vi "OrdenarPosZagueiros.vi"(9 "geometry":T1, 11 "IA State Input 2":T2={"our_robots"=[], "enemy_robots"=[], "balls"=[], "geometry"={"line_width"=0, "field_length"=0, "field_width"=0, "boundary_width"=0, "referee_width"=0, "goal_width"=0, "goal_depth"=0, "goal_wall_width"=0, "center_circle_radius"=0, "defense_radius"=0, "defense_stretch"=0, "free_kick_from_defense_dist"=0, "penalty_spot_from_field_line_dist"=0, "penalty_line_from_spot_dist"=0}, "IA Judge"={"stage"="", "command"="", "our_goalie_id"=0.0, "enemy_goalie_id"=0.0, "command enum"=enum."Halt", "Time"=enum."Azul"}, "Received Timestamp"=timestamp(0 s since 1904-01-01), "Events"={"Touch"=FALSE, "Ball out"=FALSE, "id touch"=0.0, "Ball out of \nVision"=FALSE, "Ball inside \nGoalie area"=FALSE, "Robot not responding"=FALSE, "Robots responding status"=[1.0, 1.0, 1.0, 1.0, 1.0, 1.0], "Enemy Ball \nPossession"=FALSE, "Pass State"=FALSE, "id end of pass"=0.0, "Kick"=FALSE, "Id ini Possession"=0.0, "Ball Possesion"=FALSE, "Id Possesion"=0.0}}) -> (1 "Pos ordenana zagueiro 3":dbl[](array[numeric]) format="%#_13g", 2 "Pos ordenana zagueiro 2":dbl[](array[numeric]) format="%#_13g", 3 "Pos ordenana zagueiro 1":dbl[](array[numeric]) format="%#_13g")   [LabVIEW 2017]
uses:
  Core/AI Input.ctl
  Core/AI Robot.ctl
  Functions Enum.ctl
  AttackerStates.ctl
  Path Planning/RRT/PathDests.ctl
  Path Planning/RRT/PathDest.ctl
  Core/AI Ball.ctl
  Core/Field Size.ctl
  Core/AI Judge.ctl
  Command Enum.ctl
  Util/Events/Events.ctl
  b2e2cdbb-412d-44fb-bdeb-310cb0e881f7.vi
  75349cc0-a444-4d38-b1df-a3230ebe8c70.vi
  <vilib>/Array/Sort 2D Array - Pop Stack.vi
  <vilib>/Array/Sort 2D Array - Push Stack.vi
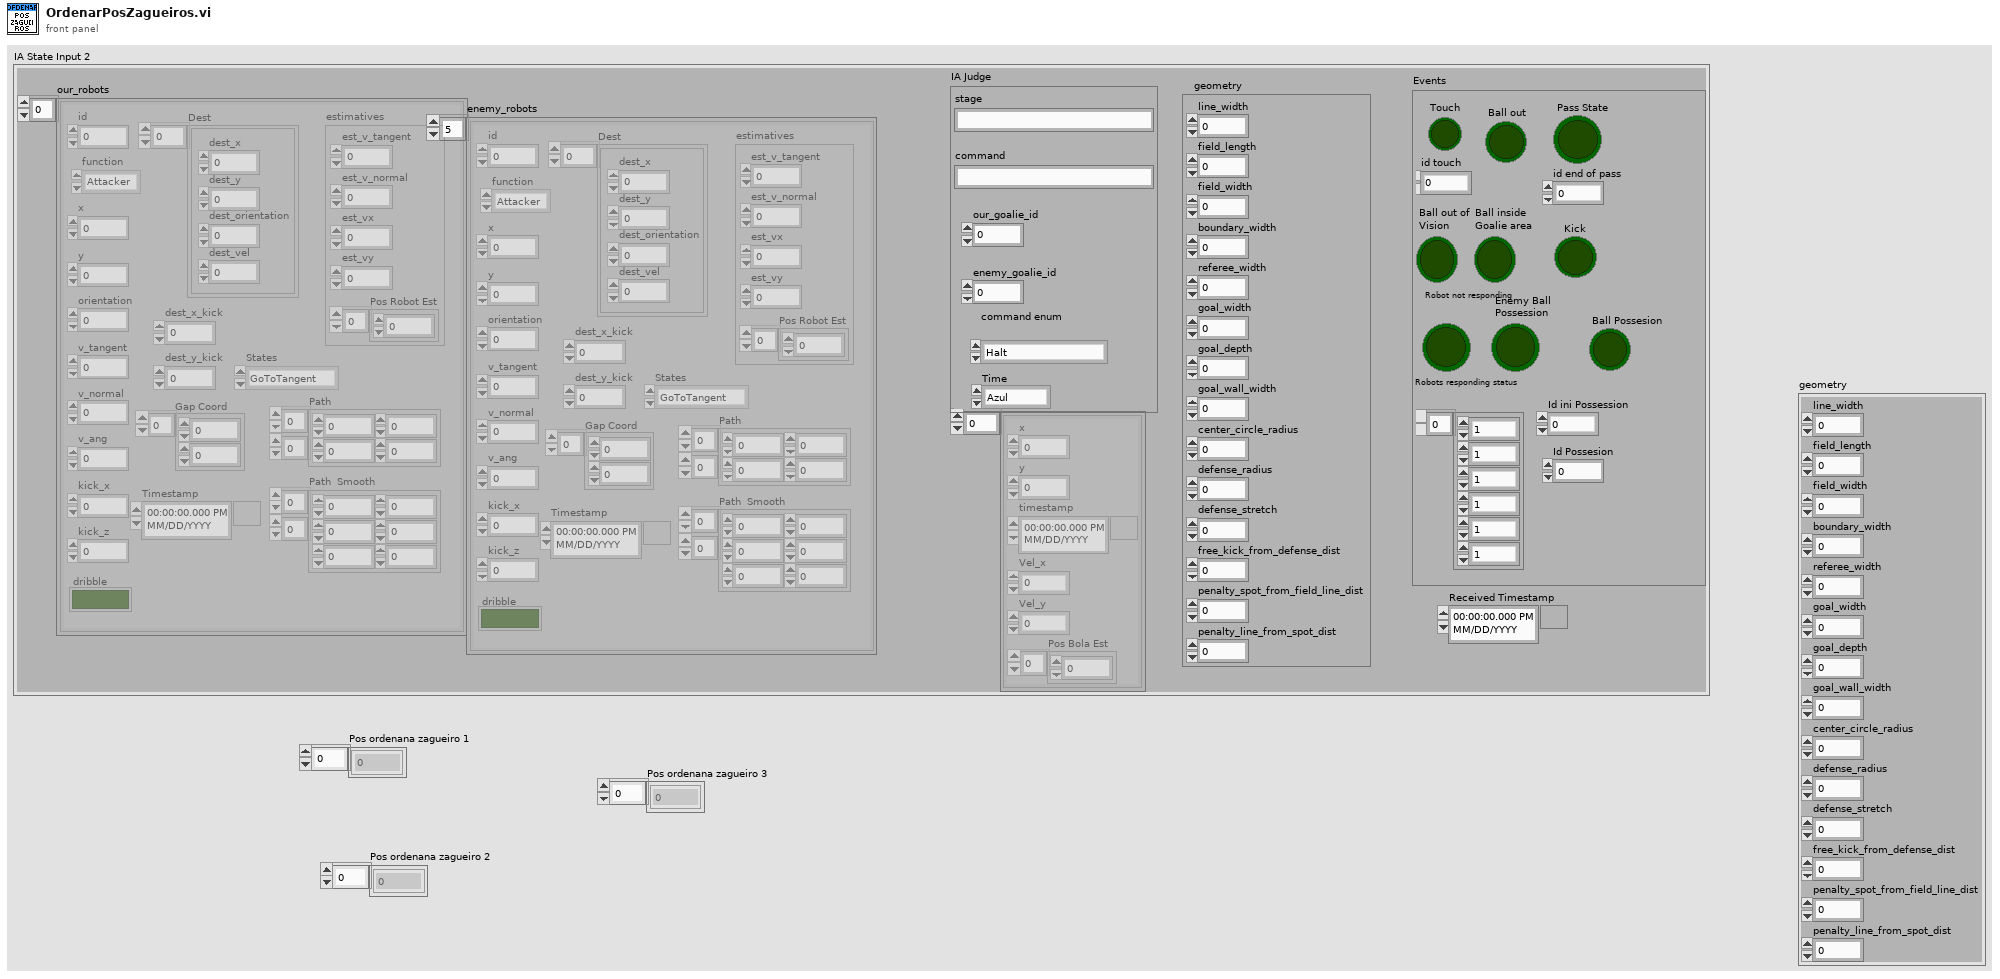
[diagram p1: front panel]
types:
  T1 = typedef "Field Size.ctl" = cluster{"line_width":u32, "field_length":u32, "field_width":u32, "boundary_width":u32, "referee_width":u32, "goal_width":u32, "goal_depth":u32, "goal_wall_width":u32, "center_circle_radius":u32, "defense_radius":u32, "defense_stretch":u32, "free_kick_from_defense_dist":u32, "penalty_spot_from_field_line_dist":u32, "penalty_line_from_spot_dist":u32}
  T2 = typedef "AI Input.ctl" = cluster{"our_robots":T3[], "enemy_robots":T3[], "balls":T8[], "geometry":T1, "IA Judge":T9, "Received Timestamp":timestamp, "Events":T11}
  T3 = typedef "AI Robot.ctl" = cluster{"id":u32, "function":T4, "x":dbl, "y":dbl, "orientation":dbl, "v_tangent":dbl, "v_normal":dbl, "v_ang":dbl, "kick_x":dbl, "kick_z":dbl, "dribble":bool, "Timestamp":timestamp, "estimatives":cluster{"est_v_tangent":dbl, "est_v_normal":dbl, "est_vx":dbl, "est_vy":dbl, "Pos Robot Est":dbl[]}, "dest_x_kick":dbl, "dest_y_kick":dbl, "Gap Coord":dbl[], "States":T5, "Path ":dbl[][], "Path  Smooth":dbl[][], "Dest":T6}
  T4 = typedef "Functions Enum.ctl" = enum16{"Attacker", "Goalie", "Defender", "Striker", "Goto 0", "Dummy", "Kicker", "ZigZag"}
  T5 = typedef "AttackerStates.ctl" = enum16{"Pass", "GoToTangent", "BallGetting", "GoToKick", ""}
  T6 = typedef "PathDests.ctl" = T7[]
  T7 = typedef "PathDest.ctl" = cluster{"dest_x":dbl, "dest_y":dbl, "dest_orientation":dbl, "dest_vel":dbl}
  T8 = typedef "AI Ball.ctl" = cluster{"x":dbl, "y":dbl, "timestamp":timestamp, "Vel_x":dbl, "Vel_y":dbl, "Pos Bola Est":dbl[]}
  T9 = typedef "AI Judge.ctl" = cluster{"stage":string, "command":string, "our_goalie_id":dbl, "enemy_goalie_id":dbl, "command enum":T10, "Time":enum16{"Azul", "Amarelo"}}
  T10 = typedef "Command Enum.ctl" = enum16{"Halt", "Stop", "Force Start", "PKA Normal Start", "Prepare Kickoff Ally", "PKE Normal Start", "Prepare Kickoff Enemy", "Prepare Penalty Ally", "PPA Normal Start", "Prepare Penalty Enemy", "PPE Normal Start", "Direct Free Enemy", "Direct Free Ally", "Indirect Free Enemy", "Indirect Free Ally", "Timeout Enemy", "Timeout Ally", "Goal Enemy", "Goal Ally", "Ball Placement Enemy", "Ball Placement Ally", "Normal Half Time", "Extra Time Break", "Extra Half Time", "None", "Post Game"}
  T11 = typedef "Events.ctl" = cluster{"Touch":bool, "Ball out":bool, "id touch":dbl, "Ball out of \nVision":bool, "Ball inside \nGoalie area":bool, "Robot not responding":bool, "Robots responding status":dbl[], "Enemy Ball \nPossession":bool, "Pass State":bool, "id end of pass":dbl, "Kick":bool, "Id ini Possession":dbl, "Ball Possesion":bool, "Id Possesion":dbl}
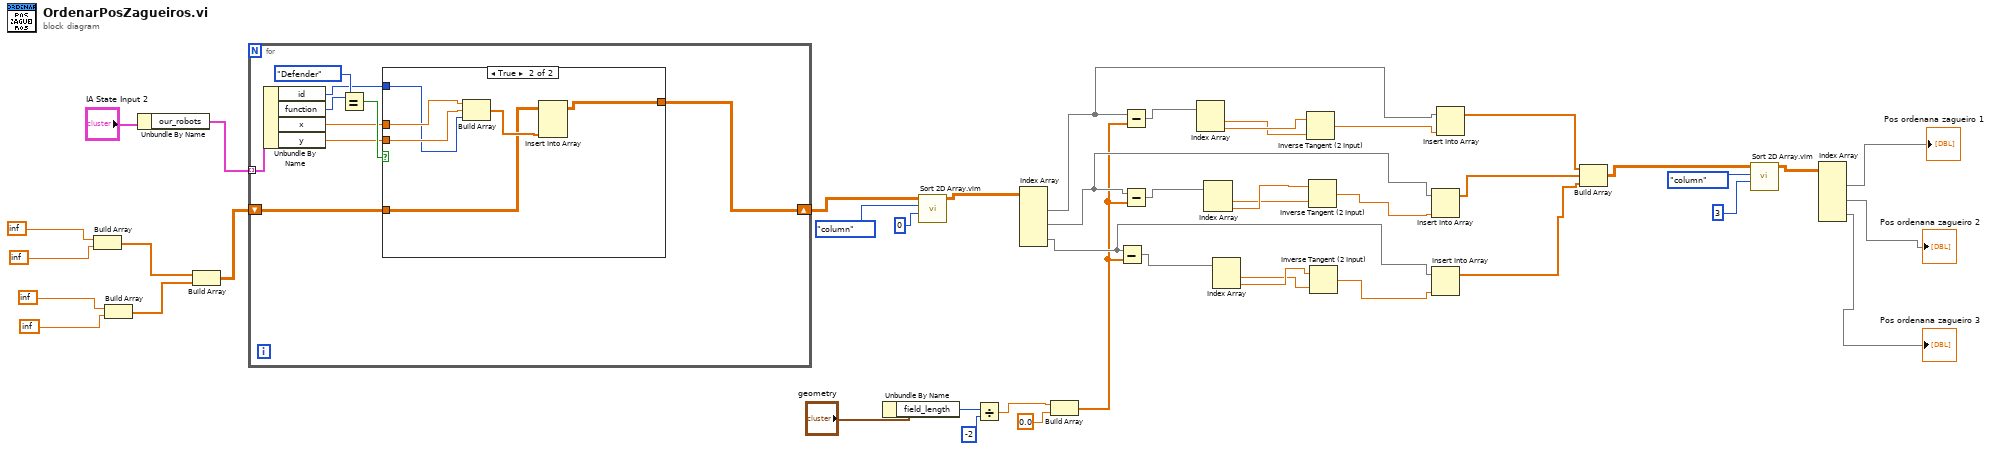
[diagram p0: block diagram]
diagram:
  n1 = Build Array(inf, inf) -> (w38:dbl[])
  n2 = Build Array(inf, inf) -> (w37:dbl[])
  n3 = Unbundle By Name("IA State Input 2") -> ("our_robots"=w43:T3[])
  n4 = Build Array(w38, w37) -> (w36:dbl[][])
  n5 = for {
    tunnel: w43 -> [w53] mode=indexing
    shift-right: [w46] -> w35
    shift-left: w36 -> [w45]
    n6 = Unbundle By Name(w53) -> ("id"=w47:u32, "function"=w52:T4, "x"=w49:dbl, "y"=w48:dbl)
    n7 = Equal?(x=w52, y=Functions_Enum."Defender") -> (x = y?=w50:bool)
    n8 = case shown="True" w50 {
      tunnel: w49 -> [_ w60]
      tunnel: w48 -> [_ w59]
      tunnel: w47 -> [_ w58]
      tunnel: [w54 w56] -> w46
      tunnel: w45 -> [w54 w55]
      frame False {
      }
      frame True {
        n9 = Build Array(w60, w59, w58) -> (w57:dbl[])
        n10 = Insert Into Array(array=w55, new element=w57) -> (w56:dbl[][])  [unwired: 2 in]
      }
    }
  }
  n11 = Unbundle By Name("geometry") -> ("field_length"=w30:u32)
  n12 = call "Sort 2D Array.vim"("index"=0, "dimension to index (column)"=enum16{"column", "row"}."column", "2D array"=w35) -> ("sorted 2D array"=w32:dbl[][])  [unwired: 7 in, 1 out]
  n13 = Divide(x=w30, y=-2) -> (x/y=w28:dbl)
  n14 = Index Array(array=w32) -> (element #1=w17:dbl[], element #2=w15:dbl[], element #3=w13:dbl[])  [unwired: 6 in]
  n15 = Build Array(w28, 0.0 ("element")) -> (w1:dbl[])
  n16 = Subtract(x=w13, y=w1) -> (x-y=w24:dbl[])
  n17 = Subtract(x=w17, y=w1) -> (x-y=w26:dbl[])
  n18 = Subtract(x=w15, y=w1) -> (x-y=w25:dbl[])
  n19 = Index Array(array=w26) -> (element #1=w22:dbl, element #2=w23:dbl)  [unwired: 2 in]
  n20 = Index Array(array=w25) -> (element #1=w20:dbl, element #2=w21:dbl)  [unwired: 2 in]
  n21 = Index Array(array=w24) -> (element #1=w18:dbl, element #2=w19:dbl)  [unwired: 2 in]
  n22 = Inverse Tangent (2 Input)(1:w22, 2:w23) -> (0:w16:dbl)
  n23 = Inverse Tangent (2 Input)(1:w20, 2:w21) -> (0:w14:dbl)
  n24 = Inverse Tangent (2 Input)(1:w18, 2:w19) -> (0:w12:dbl)
  n25 = Insert Into Array(array=w15, new element=w14) -> (w10:dbl[])  [unwired: 1 in]
  n26 = Insert Into Array(array=w13, new element=w12) -> (w9:dbl[])  [unwired: 1 in]
  n27 = Insert Into Array(array=w17, new element=w16) -> (w11:dbl[])  [unwired: 1 in]
  n28 = Build Array(w11, w10, w9) -> (w8:dbl[][])
  n29 = call "Sort 2D Array.vim"("index"=3, "dimension to index (column)"=enum16{"column", "row"}."column", "2D array"=w8) -> ("sorted 2D array"=w5:dbl[][])  [unwired: 7 in, 1 out]
  n30 = Index Array(array=w5) -> (element #1=→"Pos ordenana zagueiro 1":dbl[], element #2=→"Pos ordenana zagueiro 2":dbl[], element #3=→"Pos ordenana zagueiro 3":dbl[])  [unwired: 6 in]
